vi "Get_Counter.vi"(8 "error in (no error)":errorcluster, 10 "Number of Measurements (1) in":i32, 11 "VISA Refnum in":refnum<visa-resource-name>) -> (0 "error out":errorcluster, 2 "Numeric":dbl, 3 "VISA Refnum out":refnum<visa-resource-name>)   [LabVIEW 2013]
uses:
  <vilib>/Analysis/baseanly.llb/Mean (DBL).vi
  <instrlib>/Tektronix FCA MCA 3000 Series/Public/Data/Read Measurement (Multiple).vi
  <instrlib>/Tektronix FCA MCA 3000 Series/Tektronix FCA MCA 3000 Series.lvlib
  <vilib>/Analysis/NI_AALBase.lvlib
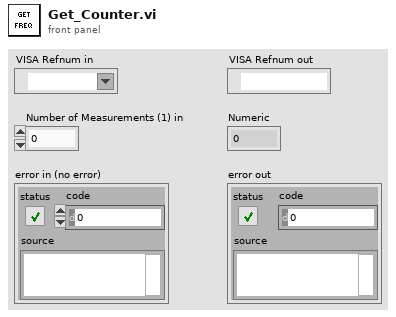
[diagram p1: front panel]
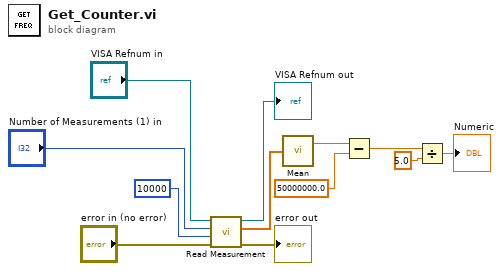
[diagram p0: block diagram]
diagram:
  n1 = call-poly <instrlib>:"Read Measurement.vi"("error in (no error)"="error in (no error)", "Timeout (10000 ms)"=10000, "Number of Measurements (1)"="Number of Measurements (1) in", "VISA resource name"="VISA Refnum in") -> ("error out"=→"error out":errorcluster, "Measurements"=w3:ext[], "VISA resource name out"=→"VISA Refnum out":refnum<visa-resource-name>)  [unwired: 5 in]
  n2 = call-poly <vilib>:"Mean.vi"("X"=w3) -> ("mean"=w2:dbl)  [unwired: 1 out]
  n3 = Subtract(x=w2, y=50000000.0) -> (x-y=w11:dbl)
  n4 = Divide(x=w11, y=5.0) -> (x/y=→"Numeric":dbl)
